vi "Read connections status.vi"(8 "error in (no error)":errorcluster, 11 "TCP Slave in":refnum<class "TCP Slave.lvclass">) -> (0 "error out":errorcluster, 2 "Connections":T1[](array[typedef]), 3 "TCP Slave out":refnum<class "TCP Slave.lvclass">)   [LabVIEW 2013, in "Modbus Library - Advance.lvlib" / "TCP Slave.lvclass"]
uses:
  TCP Slave.lvclass
  Connection.ctl
  TCP Slave.lvclass/TCP Slave.ctl
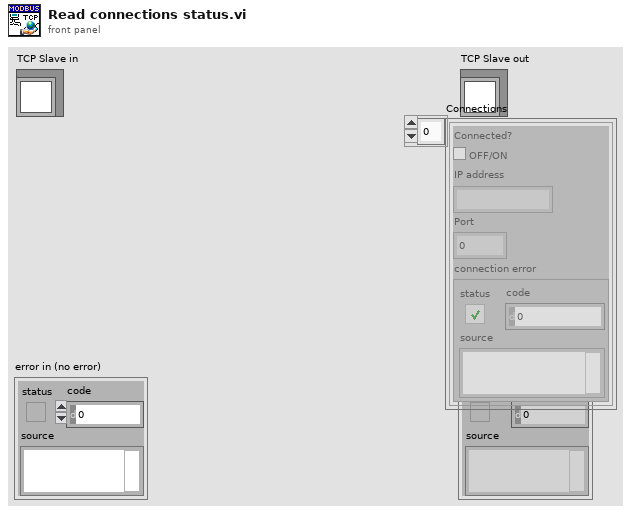
[diagram p1: front panel]
types:
  T1 = typedef "Modbus Library - Advance.lvlib/TCP Slave.lvclass/Connection.ctl" = cluster{"Connected?":bool, "IP address":string, "Port":u16, "connection error":errorcluster}
  T2 = typedef "K2Labs Modbus Library.lvlib/TCP Slave.lvclass/Connection Counter.ctl" = cluster{"Currently Connected":u32, "Connection Records":refnum<data-value>[]}
  T3 = typedef "K2Labs Modbus Library.lvlib/TCP Slave.lvclass/Connection.ctl" = cluster{"Connected?":bool, "IP address":string, "Port":u16, "connection error":errorcluster}
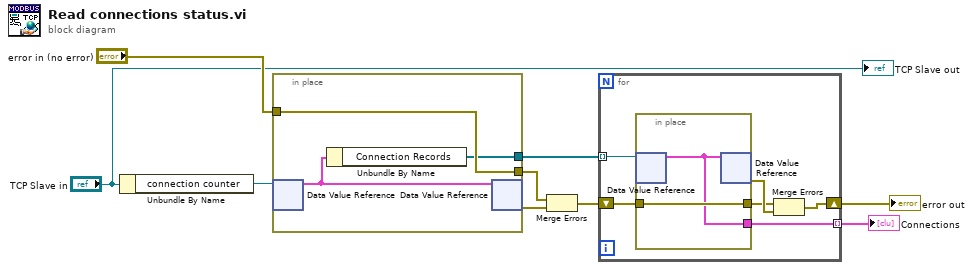
[diagram p0: block diagram]
diagram:
  n1 = Unbundle By Name("TCP Slave in") -> ("connection counter"=w5:refnum<data-value>)
  n2 = in-place {
    in-place-border: "error in (no error)" -> [w12]
    in-place-border: [w12] -> w6
    in-place-border: [w10] -> w4
    n3 = in-place-dvr #1(w5) -> (w11:T2)  [unwired: 1 out]
    n4 = Unbundle By Name(w11) -> ("Connection Records"=w10:refnum<data-value>[])
    n5 = in-place-dvr #1(w11) -> (w7:errorcluster)  [unwired: 1 out]
  }
  n6 = Merge Errors(w6, w7) -> (w3:errorcluster)
  n7 = for {
    tunnel: w4 -> [w18] mode=indexing
    shift-right: [w17] -> w2
    shift-left: w3 -> [w16]
    tunnel: [w13] -> w1 mode=indexing
    n8 = in-place {
      in-place-border: w16 -> [w20]
      in-place-border: [w20] -> w14
      in-place-border: [w19] -> w13
      n9 = in-place-dvr #2(w18) -> (w19:T3)  [unwired: 1 out]
      n10 = in-place-dvr #2(w19) -> (w15:errorcluster)  [unwired: 1 out]
    }
    n11 = Merge Errors(w14, w15) -> (w17:errorcluster)
  }
  "error out" <- w2
  "Connections" <- w1
  "TCP Slave out" <- "TCP Slave in"
